vi "getGratingPosition.vi"(6 "Delay between send and receive [ms]":i32=100, 8 "error in (no error)":errorcluster, 11 "Monochromator in":refnum<class "Monochromator.lvclass">) -> (0 "error out":errorcluster, 2 "position":i32, 3 "Monochromator out":refnum<class "Monochromator.lvclass">)   [LabVIEW 2023, in "Monochromator.lvclass"]
doc: "Returns the current grating turret position.\n\nNote: Prior to the initialization of the grating turret, this value may not reflect the actual position of the turret. To read the current position of the grating turret, please run mono_init prior to running this command."
uses:
  Monochromator.lvclass
  GratingPosition.ctl
  d9b87029-586e-44ee-a6e5-d4a5e0edce38.vi
  b59fd1e7-dcda-425c-bd6c-61aafb79e7f4.vi
  <vilib>/JDP Science/JSONtext/Variant to JSON Text.vi
  <vilib>/JDP Science/JSONtext/Set Item.vi
  <vilib>/JDP Science/JSONtext/JSON text to Variant.vi
  <vilib>/JDP Science/JSONtext/LVClass Serializer/JSONtext LVClass Serializer.lvclass
  Monochromator.lvclass/Monochromator.ctl
  GenericDevice/GenericDevice.lvclass
  <vilib>/JDP Science/JSONtext/JSONtext.lvlib
panel:
  # "Connector Pane"
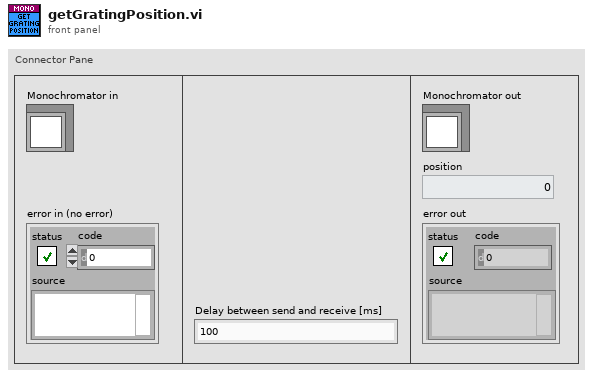
[diagram p1: front panel]
types:
  T1 = typedef "Monochromator.lvclass/GratingPosition.ctl" = cluster{"position":i32}
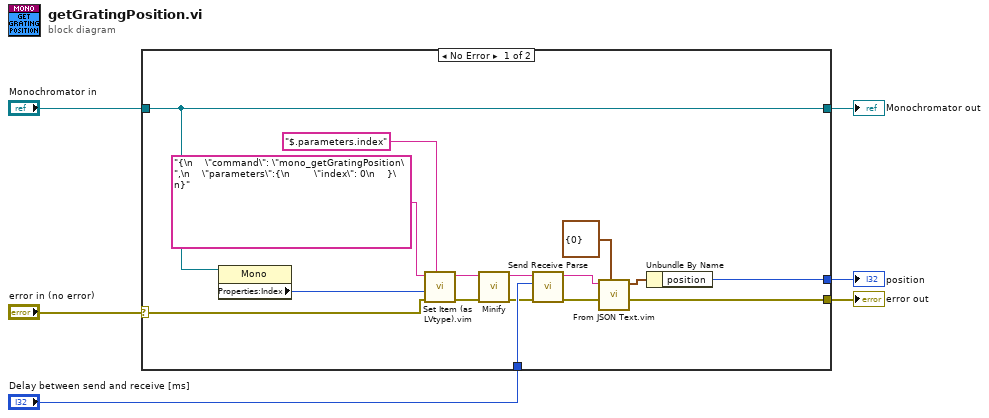
[diagram p0: block diagram]
diagram:
  n1 = case shown="No Error" "error in (no error)" {
    selector: "error in (no error)" -> [w18 w24]
    tunnel: [w17 w24] -> w5
    tunnel: [w20 w23] -> w3
    tunnel: "Monochromator in" -> [w20 w23]
    tunnel: [w12 _] -> w2
    tunnel: "Delay between send and receive [ms]" -> [w10 _]
    frame No Error {
      n2 = property class="Mono"(reference=w20) -> ("Properties:Index"=w19:i32)  [unwired: 1 in, 2 out]
      n3 = call "Set Item (as LVtype).vim"("$Path or Item Name"="$.parameters.index", "error in (no error)"=w18, "Anything"=w19, "JSON"="{\n    \"command\": \"mono_getGratingPosition\",\n    \"parameters\":{\n        \"index\": 0\n    }\n}") -> ("error out"=w16:errorcluster, "<JSON>"=w8:string)  [unwired: 4 in, 1 out]
      n4 = call <vilib>:"Minify.vi"("error in (no error)"=w16, "JSON"=w8) -> ("error out"=w9:errorcluster, "<JSON>"=w7:string)  [unwired: 7 in, 1 out]
      n5 = call "Send Receive Parse.vi"("error in"=w9, "Delay between send and receive [ms]"=w10, "<JSON>"=w7) -> ("error out"=w14:errorcluster, "results-JSON string"=w15:string)  [unwired: 6 in, 1 out]
      n6 = call "From JSON Text.vim"("Data Type and Default Value"=T1 {"position"=0} ("Grating Position"), "error in (no error)"=w14, "JSON"=w15) -> ("error out"=w17:errorcluster, "Data out"=w13:T1)  [unwired: 7 in]
      n7 = Unbundle By Name(w13) -> ("position"=w12:i32)
    }
    frame Error {
    }
  }
  "error out" <- w5
  "Monochromator out" <- w3
  "position" <- w2
